vi "Set Voltage.vi"(7 "Voltage Param (amplitude)":T1, 8 "error in (no error)":errorcluster, 9 "voltage":dbl[unit], 10 "Channel (0: Channel 1)":T2 items=["Channel 1", "Channel 2"], 11 "VISA resource name":refnum<visa-resource-name>) -> (0 "error out":errorcluster, 3 "VISA resource name out":refnum<visa-resource-name>)   [LabVIEW 2015, in "Tektronix AFG 3000 Series.lvlib"]
doc: "Sets the voltage of a Tektronix AFG 3000 series function generator; used for setting high, low, offset, or amplitude, as well as high and low voltage limits. <B>Note:</B> depending on which voltage you're setting and what the voltage units are set for (default: VPP), you may be setting volts peak to peak, volts RMS, or even DBM."
uses:
  Tektronix AFG 3000 Series.lvlib
  controls.llb/Channel.ctl
  controls.llb/Voltage.ctl
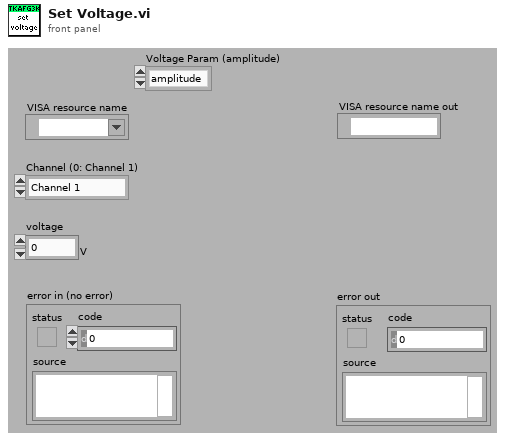
[diagram p1: front panel]
types:
  T1 = typedef "Voltage.ctl" = enum16{"amplitude", "offset", "high", "low", "high limit", "low limit"}
  T2 = typedef "Channel.ctl" = u16
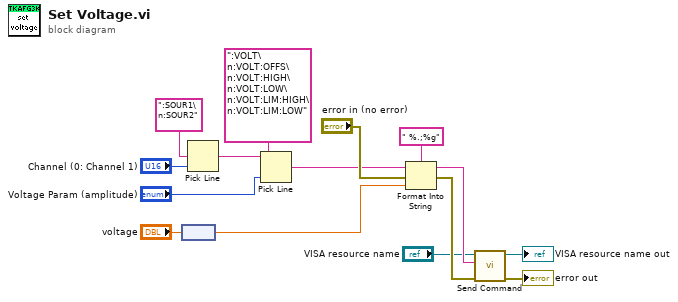
[diagram p0: block diagram]
diagram:
  n1 = node("voltage") -> (w4:dbl)
  n2 = Pick Line(multi-line string=":SOUR1\n:SOUR2", line index="Channel (0: Channel 1)") -> (output string=w8:string)  [unwired: 1 out]
  n3 = Pick Line(string ("")=w8, multi-line string=":VOLT\n:VOLT:OFFS\n:VOLT:HIGH\n:VOLT:LOW\n:VOLT:LIM:HIGH\n:VOLT:LIM:LOW", line index="Voltage Param (amplitude)") -> (output string=w5:string)
  n4 = Format Into String(format string=" %.;%g", initial string=w5, error in="error in (no error)", w4) -> (resulting string=w12:string, error out=w10:errorcluster)
  n5 = call "Send Command.vi"("error in (no error)"=w10, "write buffer"=w12, "VISA resource name"="VISA resource name") -> ("error out"=→"error out":errorcluster, "VISA resource name out"=→"VISA resource name out":refnum<visa-resource-name>)  [unwired: 7 out]
